vi "Circle0001.vi"   [LabVIEW 2013]
uses:
  <vilib>/Heliosphere Research LLC/Advanced Plotting Toolkit/typedefs/PlotID.ctl
  ErrorCodes.ctl
  <vilib>/Heliosphere Research LLC/Advanced Plotting Toolkit/Advanced Plotting Toolkit.lvlib
types:
  T1 = typedef "ErrorCodes.ctl" = u32
  T2 = typedef "Advanced Plotting Toolkit.lvlib/PlotID.ctl" = i32
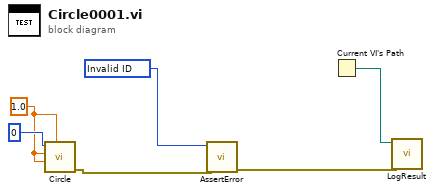
[diagram p0: block diagram]
diagram:
  w1 = T1 402902 items=["Invalid ID"=402902, "Failed to Init"=402900, "Unknown Error"=402901, "Save - Bad File Extension"=402403, "Save - General Error"=402904, "Unsupported (Polar)"=402905, "Unsupported (Logscale)"=402906, "Coordinates Not Regular"=402907] ("Error Codes")
  w2 = 1.0 ("X Position")
  n1 = call <vilib>:"Circle.vi"("Radius"=w2, "Y Position"=w2, "X Position"=w2, "Plot ID"=T2 0 ("Plot ID In")) -> ("error out"=w3:errorcluster)  [unwired: 6 in, 1 out]
  n2 = call "AssertError.vi"("error in (no error)"=w3, "Expected Error"=w1) -> ("error out"=w5:errorcluster)  [unwired: 9 in]
  n3 = Current VI's Path() -> (path=w6:path)
  n4 = call "LogResult.vi"("Test Result"=w5, "VI Path"=w6) -> ()  [unwired: 10 in]
